vi "cảm biến nhiệt độ.vi"() -> ()   [LabVIEW 2020]
uses:
  <vilib>/LabVIEW Interface for Arduino/Type Defs/Board Type.ctl
  <vilib>/LabVIEW Interface for Arduino/Type Defs/Connection Type.ctl
  <vilib>/LabVIEW Interface for Arduino/Type Defs/Pin Mode.ctl
  <vilib>/LabVIEW Interface for Arduino/LabVIEW Interface for Arduino.lvlib
panel:
  in  "Board Type (Uno)":T1
  in  "Analog Input Pin (0)":u8
  in  "stop":bool
  out "Boolean":bool
  in  "gia tri dat":dbl
  out "Waveform Chart":dbl(graph)
  out "Thermometer":dbl(slide) scale=0.0..100.0
  in  "VISA resource":refnum<visa-resource-name>
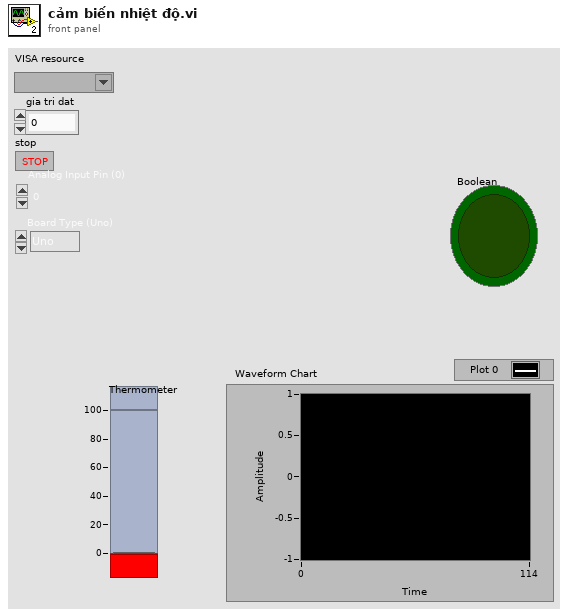
[diagram p1: front panel]
types:
  T1 = typedef "LabVIEW Interface for Arduino.lvlib/Board Type.ctl" = enum16{"Uno", "Dimuelanove w/Atmega 328", "Mega 2560"}
  T2 = typedef "LabVIEW Interface for Arduino.lvlib/Connection Type.ctl" = enum8{"USB / Serial", "XBEE", "BlueSmirf (Bluetooth)"}
  T3 = typedef "LabVIEW Interface for Arduino.lvlib/Arduino Resource.ctl" = cluster{"VISA resource":refnum<visa-resource-name>, "Board Type":T1, "Connection Type":enum8{"USB / Serial"}, "Bytes Per Packet (15)":u8}
  T4 = typedef "LabVIEW Interface for Arduino.lvlib/Pin Mode.ctl" = enum8{"Input", "Output"}
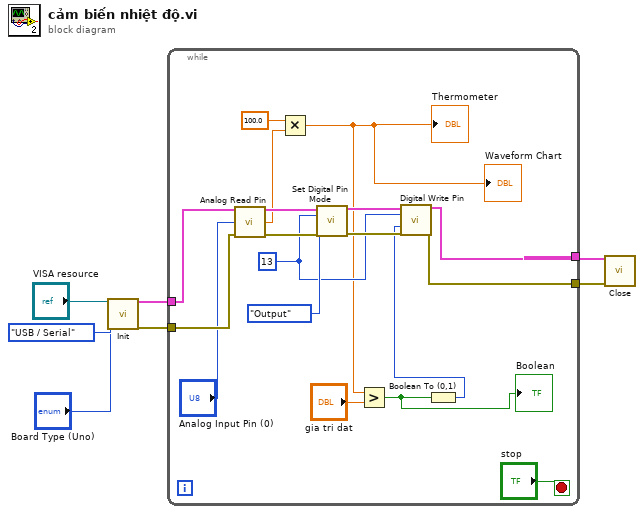
[diagram p0: block diagram]
diagram:
  n1 = call <vilib>:"Init.vi"("VISA resource"="VISA resource", "Board Type (Uno)"="Board Type (Uno)", "Connection Type (USB/Serial)"=Connection_Type."USB / Serial") -> ("Arduino Resource"=w5:T3, "error out"=w4:errorcluster)  [unwired: 15 in]
  n2 = while {
    tunnel: w5 -> [w25]
    tunnel: w4 -> [w21]
    tunnel: [w22] -> w3
    tunnel: [w18] -> w2
    stop <- "stop" stop-if-true
    w16 = u8 13 ("Digital I/O Pin")
    n3 = call <vilib>:"Analog Read Pin.vi"("Arduino Resource"=w25, "Analog Input Pin (0)"="Analog Input Pin (0)", "error in"=w21) -> ("Arduino Resource"=w24:T3, "Voltage"=w15:dbl, "error out"=w20:errorcluster)  [unwired: 10 in]
    n4 = Multiply(x=100.0, y=w15) -> (x*y=w13:dbl)
    "Thermometer" <- w13
    "Waveform Chart" <- w13
    n5 = call <vilib>:"Set Digital Pin Mode.vi"("Arduino Resource"=w24, "Digital I/O Pin"=w16, "Pin Mode (Input)"=Pin_Mode."Output", "error in"=w20) -> ("Arduino Resource"=w23:T3, "error out"=w19:errorcluster)  [unwired: 10 in]
    n6 = Greater?(x=w13, y="gia tri dat") -> (0:w10:bool)
    "Boolean" <- w10
    n7 = Boolean To (0,1)(Boolean=w10) -> (0, 1=w11:i16)
    n8 = call <vilib>:"Digital Write Pin.vi"("Arduino Resource"=w23, "Digital I/O Pin (0)"=w16, "Value (0)"=w11, "error in"=w19) -> ("Arduino Resource"=w22:T3, "error out"=w18:errorcluster)  [unwired: 10 in]
  }
  n9 = call <vilib>:"Close.vi"("Arduino Resource"=w3, "error in"=w2) -> ()  [unwired: 13 in, 1 out]
